vi "CSG info.vi"(8 "error in (no error)":errorcluster, 11 "Variant":variant) -> (0 "error out":errorcluster, 3 "child strings":string[](array[string]))   [LabVIEW 2017, in "Variant Tree API.lvlib"]
uses:
  Variant Tree/Source/Variant Tree API.lvlib
  <vilib>/Utility/Data Type/Get Numeric Information.vi
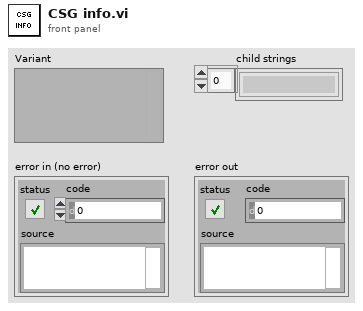
[diagram p1: front panel]
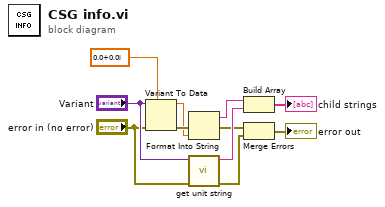
[diagram p0: block diagram]
diagram:
  n1 = Variant To Data(error in="error in (no error)", type=csg 0.0+0.0i ("Numeric"), Variant="Variant") -> (data=w3:csg, error out=w6:errorcluster)
  n2 = Format Into String(error in=w6, w3) -> (resulting string=w4:string, error out=w8:errorcluster)  [unwired: 2 in]
  n3 = call "get unit string.vi"("error in (no error)"="error in (no error)", "Variant"="Variant") -> ("error out"=w10:errorcluster, "String"=w11:string)  [unwired: 8 in]
  n4 = Build Array(w4, w11) -> (→"child strings":string[])
  n5 = Merge Errors(w8, w10) -> (→"error out":errorcluster)
